vi "Sprinkler.vi"() -> ()   [LabVIEW 8.6]
panel:
  in  "Zone Setup Array":cluster{"Zone Selector":string, "Timing":dbl}[](array[cluster])
  out "Controller Status":string
  out "Zone Indicators":T1
  in  "Water Pressure Sensor (%)":u32(slide)
  in  "Rain Sensor":bool
  in  "Run Selector":bool
  in  "Setup":bool
  in  "Start":bool
  in  "stop":bool
  # "Controls"
  # "Simulation Controls"
  # "Rain"
  # "No Rain"
  # "Continuous"
  # "Single"
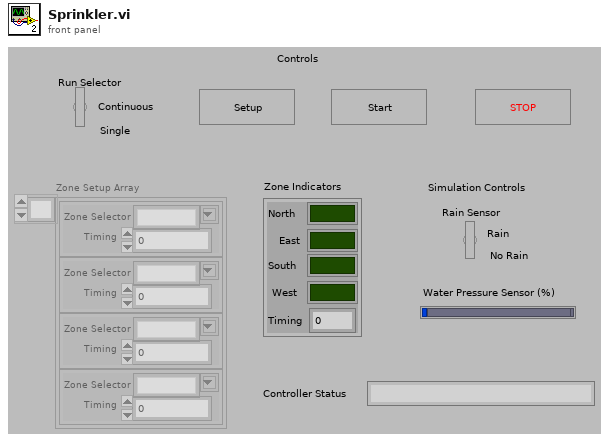
[diagram p1: front panel]
types:
  T1 = cluster{"North":bool, "East":bool, "South":bool, "West":bool, "Timing":u32}
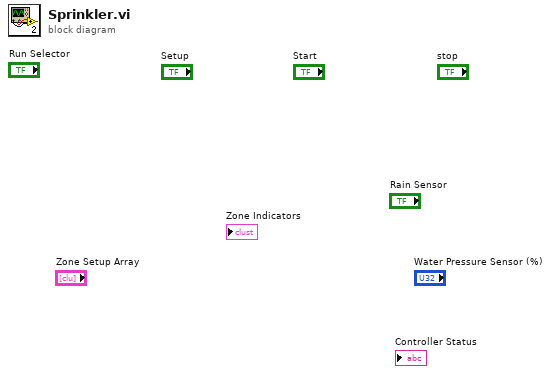
[diagram p0: block diagram]
diagram:
